vi "_FPGA_AuxPulseVoltageConvertor.vi"(9 "Amp_in":u32, 11 "PulseBases_in":u32) -> (1 "V Pulse 2":i16, 3 "V Pulse 1":i16)   [LabVIEW 2018]
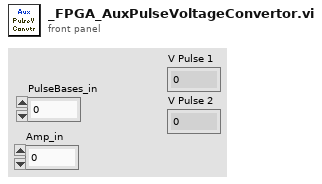
[diagram p1: front panel]
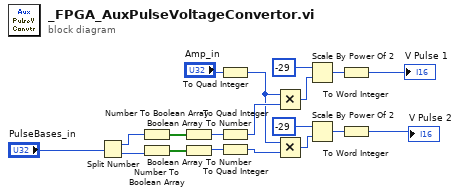
[diagram p0: block diagram]
diagram:
  n1 = Split Number(x="PulseBases_in") -> (hi(x)=w16:u16, lo(x)=w17:u16)
  n2 = Number To Boolean Array(number=w16) -> (Boolean array=w18:bool[])
  n3 = Number To Boolean Array(number=w17) -> (Boolean array=w19:bool[])
  n4 = Boolean Array To Number(Boolean array=w18) -> (number=w14:i16)
  n5 = Boolean Array To Number(Boolean array=w19) -> (number=w13:i16)
  n6 = To Quad Integer(1:"Amp_in") -> (0:w9:i64)
  n7 = To Quad Integer(1:w14) -> (0:w11:i64)
  n8 = To Quad Integer(1:w13) -> (0:w10:i64)
  n9 = Multiply(x=w9, y=w11) -> (x*y=w8:i64)
  n10 = Multiply(x=w9, y=w10) -> (x*y=w5:i64)
  n11 = Scale By Power Of 2(n=i16 -29, x=w8) -> (x*2^n=w4:i64)
  n12 = Scale By Power Of 2(n=i16 -29, x=w5) -> (x*2^n=w3:i64)
  n13 = To Word Integer(number=w4) -> (16bit integer=→"V Pulse 1":i16)
  n14 = To Word Integer(number=w3) -> (16bit integer=→"V Pulse 2":i16)
